vi "绝对偏差百分比出数.vi"(0 "基准值":dbl, 2 "原始值":dbl, 3 "绝对偏差值":dbl) -> (6 "取值输出":dbl, 7 "随机值？":bool)   [LabVIEW 2016, in "random number.lvlib"]
uses:
  random number.lvlib
panel:
  out "下限":dbl
  out "上限":dbl
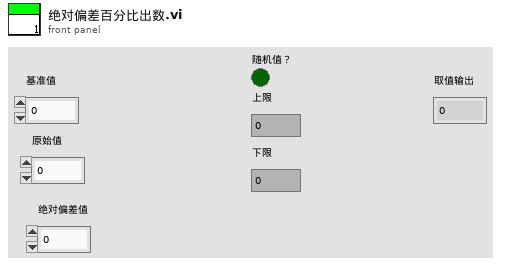
[diagram p1: front panel]
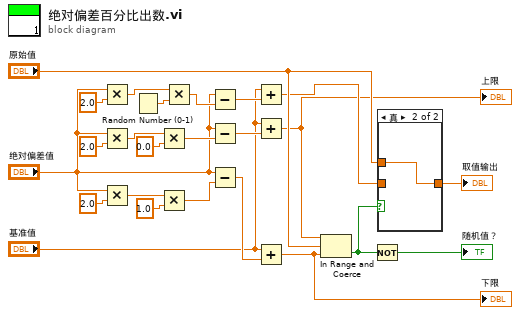
[diagram p0: block diagram]
diagram:
  n1 = Multiply(x="绝对偏差值", y=2.0) -> (x*y=w21:dbl)
  n2 = Multiply(x="绝对偏差值", y=2.0) -> (x*y=w18:dbl)
  n3 = Multiply(x="绝对偏差值", y=2.0) -> (x*y=w13:dbl)
  n4 = Random Number (0-1)() -> (number: 0 to 1=w24:dbl)
  n5 = Multiply(x=w18, y=0.0) -> (x*y=w17:dbl)
  n6 = Multiply(x=w13, y=1.0) -> (x*y=w14:dbl)
  n7 = Multiply(x=w21, y=w24) -> (x*y=w23:dbl)
  n8 = Subtract(x="绝对偏差值", y=w23) -> (x-y=w22:dbl)
  n9 = Subtract(x="绝对偏差值", y=w17) -> (x-y=w10:dbl)
  n10 = Subtract(x="绝对偏差值", y=w14) -> (x-y=w4:dbl)
  n11 = Add(x="基准值", y=w22) -> (x+y=w6:dbl)
  n12 = Add(x="基准值", y=w10) -> (x+y=w2:dbl)
  "上限" <- w2
  n13 = Add(x="基准值", y=w4) -> (x+y=w1:dbl)
  "下限" <- w1
  n14 = In Range and Coerce(upper limit=w2, x="原始值", lower limit=w1) -> (In Range?=w9:bool)  [unwired: 1 out]
  n15 = Not(x=w9) -> (.not. x?=→"随机值？":bool)
  n16 = case shown="真" w9 {
    tunnel: "原始值" -> [_ w26]
    tunnel: [w25 w26] -> w7
    tunnel: w6 -> [w25 _]
    frame False {
    }
    frame True {
    }
  }
  "取值输出" <- w7
